vi "NewMainLogLoop.vi"() -> ()   [LabVIEW 2015]
panel:
  in  "error in (no error)":errorcluster
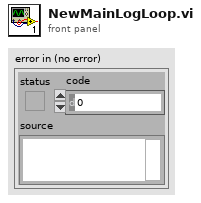
[diagram p1: front panel]
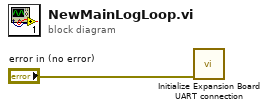
[diagram p0: block diagram]
diagram:
  n1 = call "Initialize Expansion Board UART connection.vi"("error in (no error)"="error in (no error)") -> ()  [unwired: 9 in, 2 out]
